vi "以太网自动测试.vi"(10 "选择?":bool) -> ()   [LabVIEW 2010]
uses:
  全局量/试验配置信息.vi
  全局量/自动测试结果.vi
panel:
  in  "发送数据":u32
  # "输入数据："
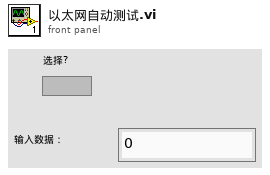
[diagram p1: front panel]
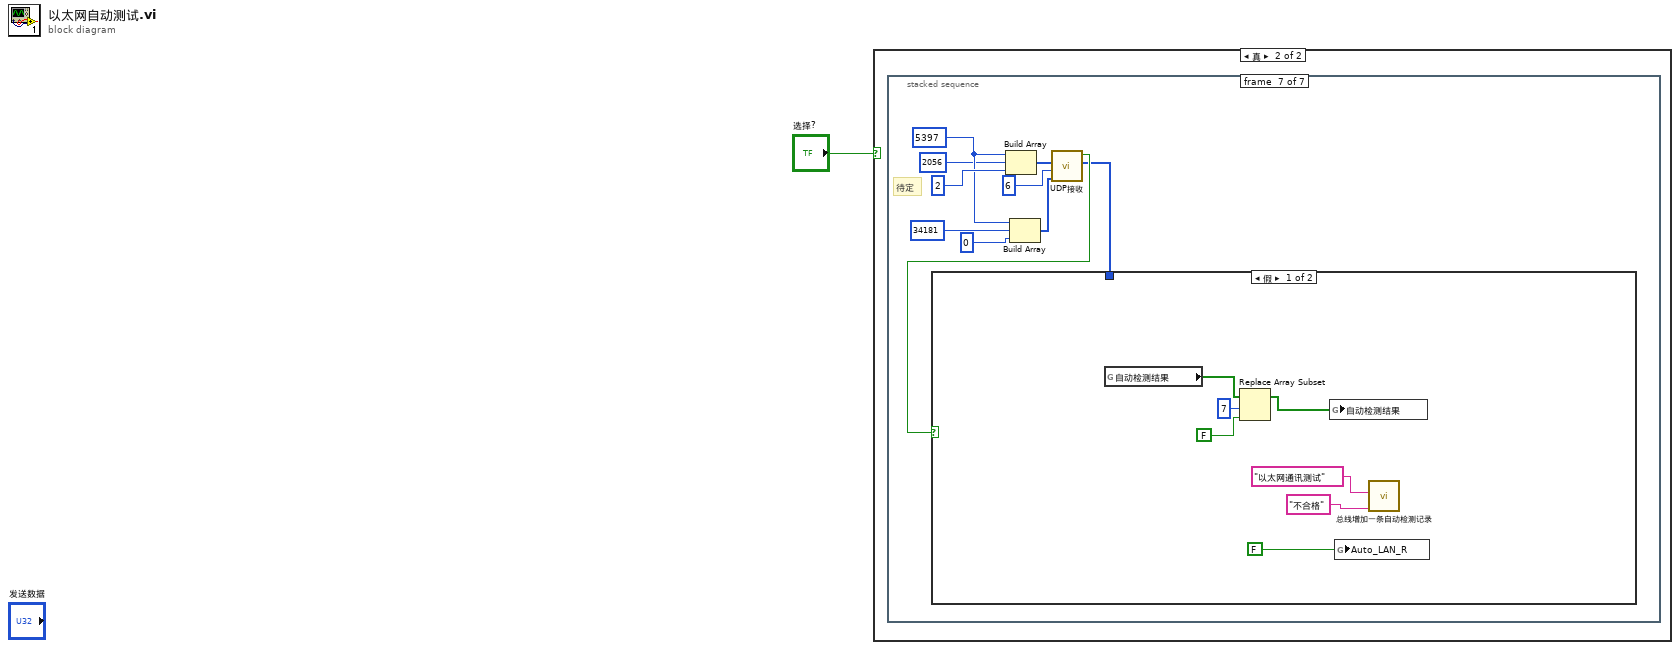
[diagram p0: block diagram]
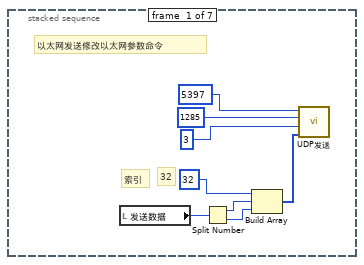
[diagram p3: hidden frame]
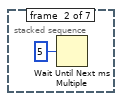
[diagram p4: hidden frame]
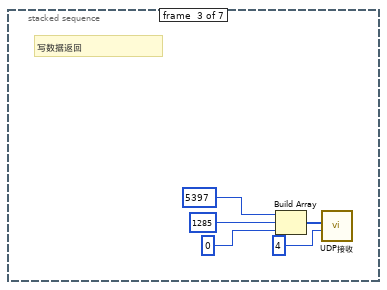
[diagram p5: hidden frame]
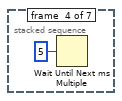
[diagram p6: hidden frame]
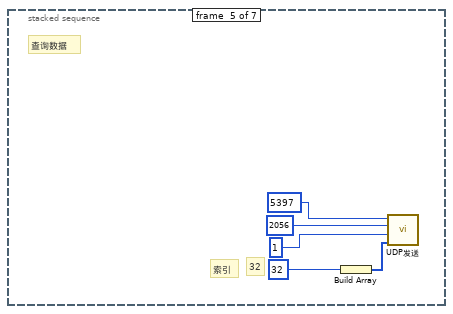
[diagram p7: hidden frame]
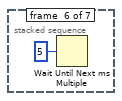
[diagram p8: hidden frame]
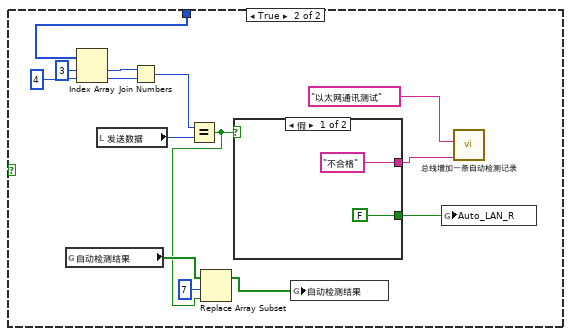
[diagram p9: hidden frame]
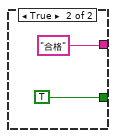
[diagram p10: hidden frame]
diagram:
  n1 = case shown="真" "选择?" {
    frame False {
    }
    frame True {
      n2 = stacked-sequence {
        frame #0 {
          # "32"
          # "以太网发送修改以太网参数命令"
          # "索引"
          n3 = local read "发送数据"() -> (w6:u32)
          n4 = Split Number(x=w6) -> (hi(x)=w4:u16, lo(x)=w3:u16)
          n5 = Build Array(u16 32, w4, w3) -> (w2:u16[])
          n6 = call "UDP发送.vi"("发送数据"=w2, "数据区字长"=u16 3, "报文类型"=u16 1285, "发送方标识"=u16 5397) -> ()  [unwired: 6 in, 1 out]
        }
        frame #1 {
          n7 = Wait Until Next ms Multiple(millisecond multiple=u32 5 ("毫秒倍数")) -> ()  [unwired: 1 out]
        }
        frame #2 {
          # "写数据返回"
          n8 = Build Array(u16 5397, u16 1285, u16 0) -> (w13:u16[])
          n9 = call "UDP接收.vi"("长度"=u16 4, "匹配帧信息_正常"=w13) -> ()  [unwired: 6 in, 4 out]
        }
        frame #3 {
          n10 = Wait Until Next ms Multiple(millisecond multiple=u32 5 ("毫秒倍数")) -> ()  [unwired: 1 out]
        }
        frame #4 {
          # "查询数据"
          # "32"
          # "索引"
          n11 = Build Array(u16 32) -> (w17:u16[])
          n12 = call "UDP发送.vi"("发送数据"=w17, "数据区字长"=u16 1, "报文类型"=u16 2056, "发送方标识"=u16 5397) -> ()  [unwired: 6 in, 1 out]
        }
        frame #5 {
          n13 = Wait Until Next ms Multiple(millisecond multiple=u32 5 ("毫秒倍数")) -> ()  [unwired: 1 out]
        }
        frame #6 {
          w29 = u16 5397
          # "待定"
          n14 = Build Array(w29, u16 2056, u16 2) -> (w27:u16[])
          n15 = Build Array(w29, u16 34181, u16 0 ("元素")) -> (w31:u16[])
          n16 = call "UDP接收.vi"("匹配帧信息_异常"=w31, "长度"=u16 6, "匹配帧信息_正常"=w27) -> ("接收的一帧数据"=w24:u16[], "正常_找到?"=w25:bool)  [unwired: 5 in, 2 out]
          n17 = case shown="假" w25 {
            tunnel: w24 -> [_ w53]
            frame False {
              n18 = global read "试验配置信息.vi" "自动检测结果"() -> (w39:bool[])
              n19 = Replace Array Subset(array=w39, new element=FALSE, index=7 ("索引")) -> (w38:bool[])
              n20 = global write "试验配置信息.vi" "自动检测结果"(w38) -> ()
              n21 = global write "自动测试结果.vi" "Auto_LAN_R"(FALSE) -> ()
              n22 = call "总线增加一条自动检测记录.vi"("测试结果"="不合格" ("Message"), "测试内容"="以太网通讯测试" ("Message")) -> ()  [unwired: 10 in]
            }
            frame True {
              n23 = global read "试验配置信息.vi" "自动检测结果"() -> (w43:bool[])
              n24 = Index Array(array=w53, index #1=3 ("索引"), index #2=4 ("索引")) -> (element #1=w48:u16, element #2=w47:u16)
              n25 = local read "发送数据"() -> (w49:u32)
              n26 = Join Numbers(hi=w48, lo=w47) -> ((hi.lo)=w50:u32)
              n27 = Equal?(x=w50, y=w49) -> (x = y?=w40:bool)
              n28 = Replace Array Subset(array=w43, new element=w40, index=7 ("索引")) -> (w42:bool[])
              n29 = case shown="假" w40 {
                tunnel: ["不合格" ("Message") "合格" ("Message")] -> w45
                tunnel: [FALSE TRUE] -> w44
                frame False {
                }
                frame True {
                }
              }
              n30 = global write "试验配置信息.vi" "自动检测结果"(w42) -> ()
              n31 = global write "自动测试结果.vi" "Auto_LAN_R"(w44) -> ()
              n32 = call "总线增加一条自动检测记录.vi"("测试结果"=w45, "测试内容"="以太网通讯测试" ("Message")) -> ()  [unwired: 10 in]
            }
          }
        }
      }
    }
  }
